vi "Simulation Lab -Sub VI - B220061.vi"() -> ()   [LabVIEW 2020]
panel:
  out "x > y? 2":bool
  out "Tank 3":dbl(slide) scale=0.0..10.0
  in  "Slide 6":dbl(slide) scale=0.0..10.0
  in  "Slide 5":dbl(slide) scale=0.0..10.0
  out "x > y?":bool
  out "Tank 2":dbl(slide) scale=0.0..10.0
  in  "Slide 4":dbl(slide) scale=0.0..10.0
  in  "Slide 3":dbl(slide) scale=0.0..10.0
  out "Tank":dbl(slide) scale=0.0..10.0
  in  "Slide 2":dbl(slide) scale=0.0..10.0
  in  "Slide":dbl(slide) scale=0.0..10.0
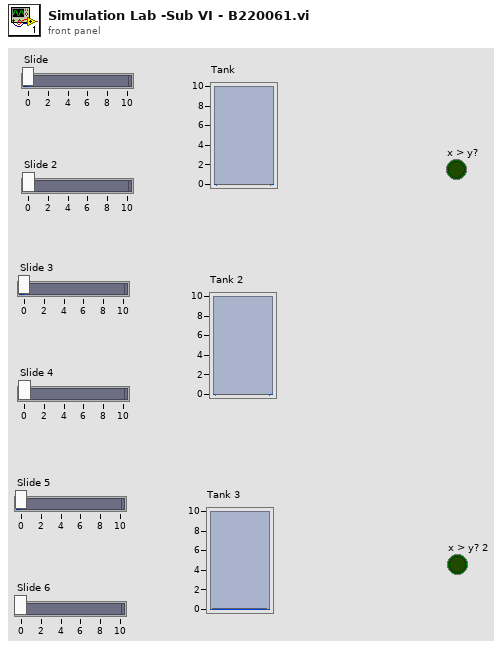
[diagram p1: front panel]
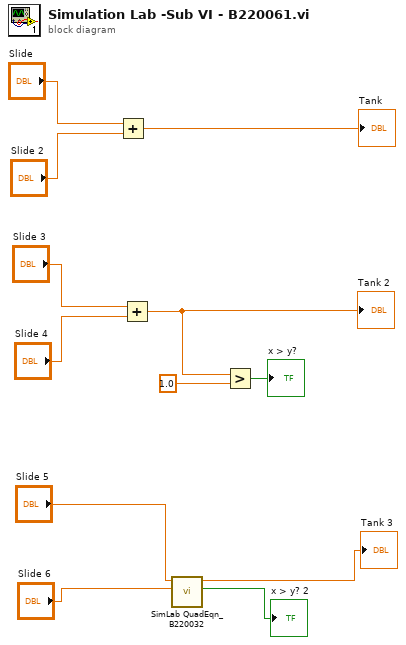
[diagram p0: block diagram]
diagram:
  n1 = Add(x="Slide", y="Slide 2") -> (x+y=→"Tank":dbl)
  n2 = Add(x="Slide 3", y="Slide 4") -> (x+y=w7:dbl)
  "Tank 2" <- w7
  n3 = call "SimLab QuadEqn_B220032.vi"("Slide 6"="Slide 6", "Slide 5"="Slide 5") -> ("x > y? 2"=→"x > y? 2":bool, "Numeric"=→"Tank 3":dbl)  [unwired: 8 in]
  n4 = Greater?(x=w7, y=1.0) -> (0:→"x > y?":bool)
